vi "Constraint.vi"(11 "UnaryOperator in":refnum<class "UnaryOperator.lvclass">) -> (2 "Constraint.lvlib:Constraint.lvclass":refnum<class "Constraint.lvclass">, 3 "UnaryOperator out":refnum<class "UnaryOperator.lvclass">)   [LabVIEW 2019, in "Constraint.lvlib" / "UnaryOperator.lvclass"]
uses:
  UnaryOperator.lvclass
  Constraint/Constraint.lvclass
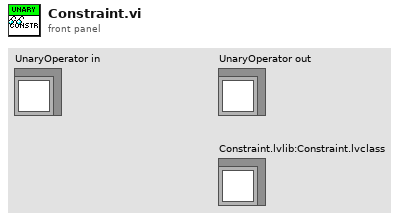
[diagram p1: front panel]
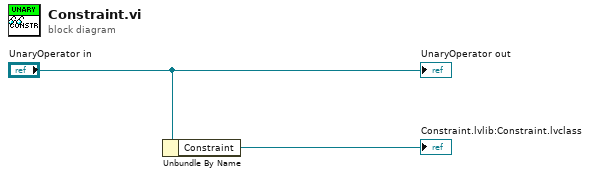
[diagram p0: block diagram]
diagram:
  n1 = Unbundle By Name("UnaryOperator in") -> ("Constraint"=→"Constraint.lvlib:Constraint.lvclass":refnum<class "Constraint.lvclass">)
  "UnaryOperator out" <- "UnaryOperator in"
